vi "week3_path-save_LV18.vi"() -> ()   [LabVIEW 2018]
uses:
  <vilib>/Utility/file.llb/Write Delimited Spreadsheet (DBL).vi
panel:
  in  "Ascii option":u16(ring) items=["Open", "Over-write", "Create", "Open or Create", "Replace or create"]
  in  "CSV_path":path
  in  "Measurement_file_path":path
  out "Numeric":dbl format="%#2.4g"
  in  "Text_path":path
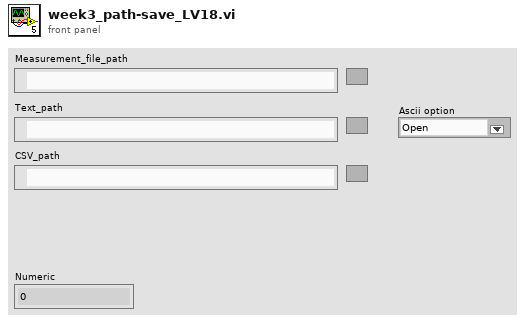
[diagram p1: front panel]
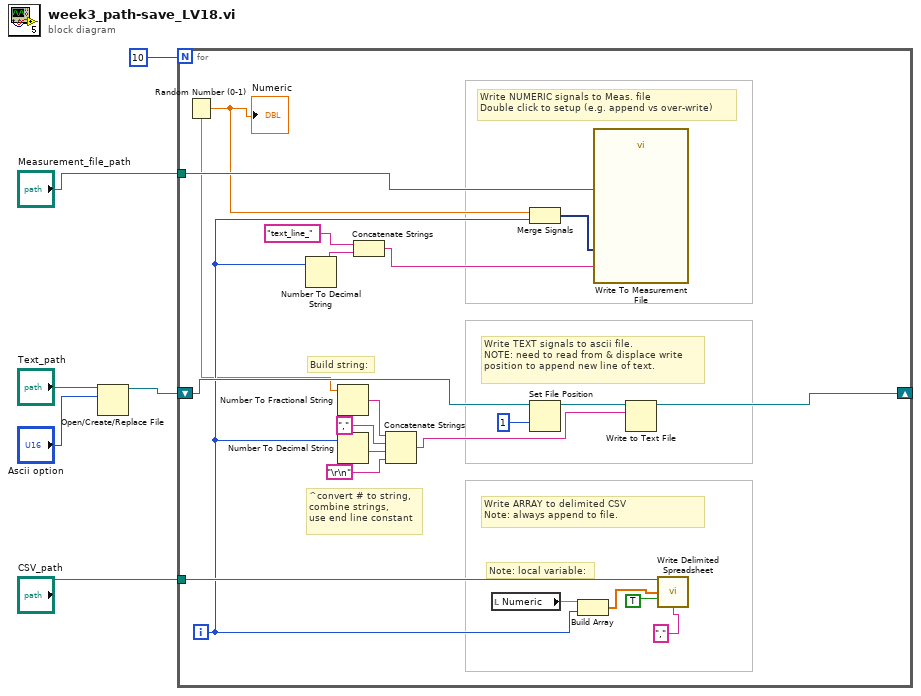
[diagram p0: block diagram]
diagram:
  n1 = Open/Create/Replace File(file path (use dialog)="Text_path", operation (0:open)="Ascii option") -> (refnum out=w4:refnum<file>)  [unwired: 4 in, 2 out]
  n2 = for {
    N: 10 -> [_]
    shift-right: [w25] -> _
    shift-left: w4 -> [w24]
    tunnel: "Measurement_file_path" -> [w21]
    tunnel: "CSV_path" -> [w17]
    i -> [w12]
    # "^convert # to string,\ncombine strings,\nuse end line constant"
    # "Build string:"
    # "Note: local variable:"
    # "Write ARRAY to delimited CSV\nNote: always append to file."
    # "Write TEXT signals to ascii file.\nNOTE: need to read from & displace write position to append new line of text."
    # "Write NUMERIC signals to Meas. file\nDouble click to setup (e.g. append vs over-write)"
    n3 = Random Number (0-1)() -> (number: 0 to 1=w11:dbl)
    "Numeric" <- w11
    n4 = Number To Decimal String(number=w12) -> (decimal integer string=w27:string)  [unwired: 1 in]
    n5 = Number To Fractional String(number=w11) -> (F-format string=w10:string)  [unwired: 3 in]
    n6 = Number To Decimal String(number=w12) -> (decimal integer string=w8:string)  [unwired: 1 in]
    n7 = Concatenate Strings("text_line_", w27) -> (w19:string)
    n8 = Concatenate Strings(w10, ",", w8, "\r\n") -> (w18:string)
    n9 = local read "Numeric"() -> (w14:dbl)
    n10 = Merge Signals(w11, w12) -> (w20:dynamicdata)
    n11 = Set File Position(refnum=w24, from (0:start)=1) -> (refnum out=w23:refnum<file>)  [unwired: 2 in, 1 out]
    n12 = Build Array(w14, w12) -> (w15:dbl[])
    n13 = call "Write To Measurement File"("Signals"=w20, "Filename"=w21, "Comment"=w19) -> ()  [unwired: 14 in, 3 out]
    n14 = Write to Text File(file (use dialog)=w23, text=w18) -> (refnum out=w25:refnum<file>)  [unwired: 2 in, 2 out]
    n15 = call-poly <vilib>:"Write Delimited Spreadsheet.vi"("file path (dialog if empty)"=w17, "1D data"=w15, "append to file? (new file:F)"=TRUE, "delimiter (\\t)"=",") -> ()  [unwired: 10 in, 2 out]
  }
